vi "罗列目录配置文件.vi"(10 "路径":path) -> (2 "数组":string[](array[string]))   [LabVIEW 2010]
panel:
  out "配置文件路径":path
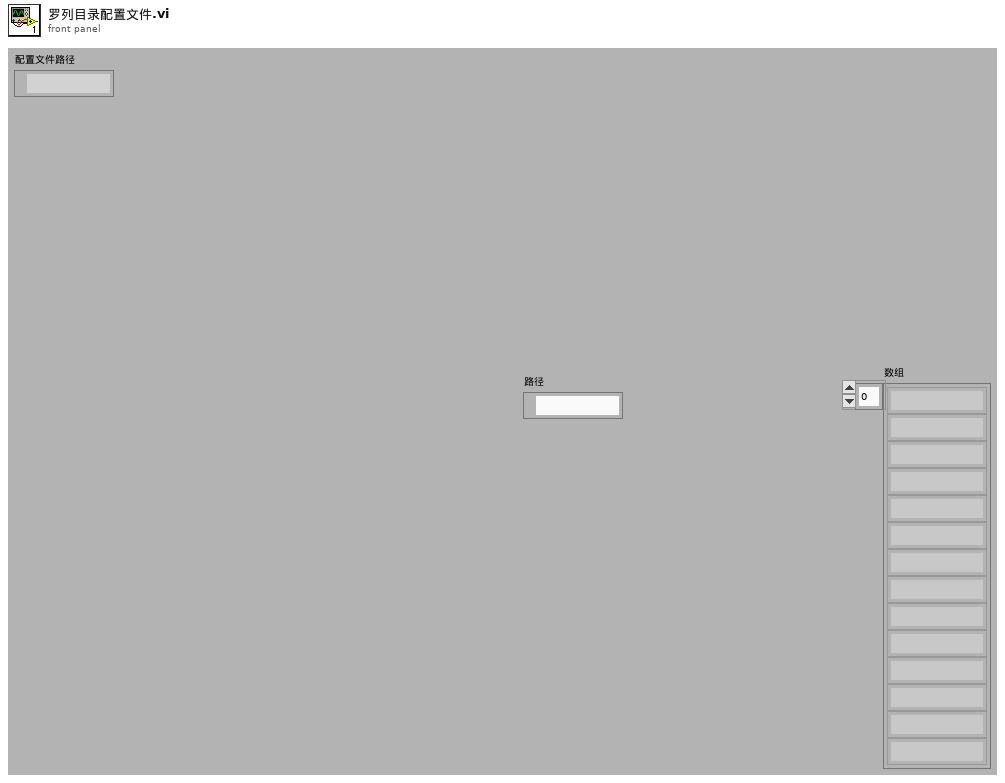
[diagram p1: front panel]
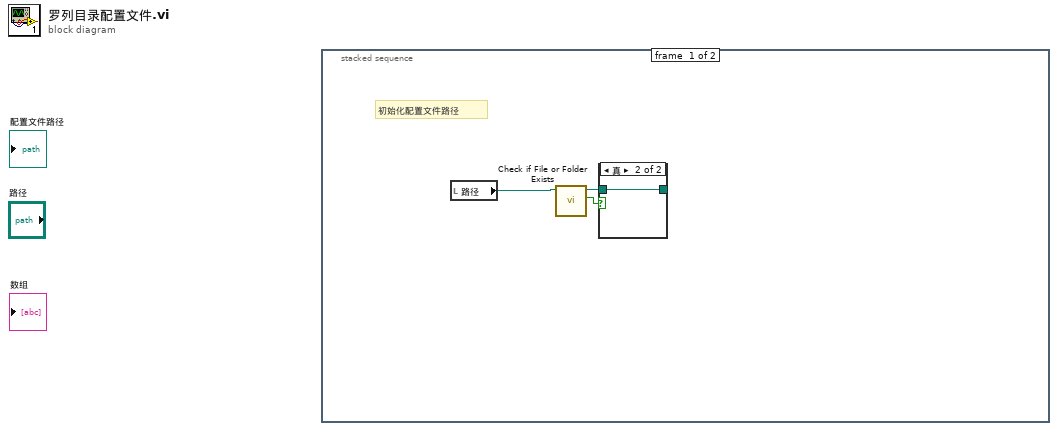
[diagram p0: block diagram]
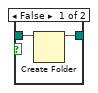
[diagram p2: hidden frame]
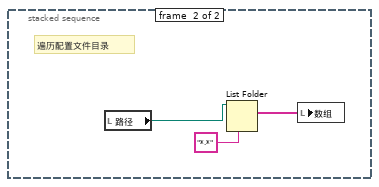
[diagram p3: hidden frame]
diagram:
  n1 = stacked-sequence {
    frame #0 {
      # "初始化配置文件路径"
      n2 = local read "路径"() -> (w1:path)
      n3 = call <vilib>:"Check if File or Folder Exists.vi"("path"=w1) -> ("file or folder exists?"=w3:bool, "dup path"=w2:path)  [unwired: 8 in, 1 out]
      n4 = case shown="真" w3 {
        tunnel: w2 -> [w5 w6]
        tunnel: [w4 w6] -> _
        frame False {
          n5 = Create Folder(path (use dialog)=w5) -> (created path=w4:path)  [unwired: 2 in, 2 out]
        }
        frame True {
        }
      }
    }
    frame #1 {
      # "遍历配置文件目录"
      n6 = local read "路径"() -> (w8:path)
      n7 = List Folder(path=w8, pattern="*.*" ("模式")) -> (filenames=w9:string[])  [unwired: 2 in, 3 out]
      n8 = local write "数组"(w9) -> ()
    }
  }
